vi "Read Counter.vi"(8 "error in (no error)":errorcluster, 10 "Params":variant, 11 "NI Counter Input in":refnum<class "NI Counter Input.lvclass">) -> (0 "error out":errorcluster, 2 "Data":variant, 3 "NI Counter Input out":refnum<class "NI Counter Input.lvclass">)   [LabVIEW 2020, in "NI DAQmx.lvlib" / "NI Counter Input.lvclass"]
uses:
  NI Counter Input.lvclass
  D:/WSGitHub/RTFWK/Realization/NI DAQmx Base/NI DAQmx Base.lvclass
  <vilib>/DAQmx/read.llb/DAQmx Read (Counter 1D DBL 1Chan NSamp).vi
  <vilib>/DAQmx/miscellaneous.llb/DAQmx Fill In Error Info.vi
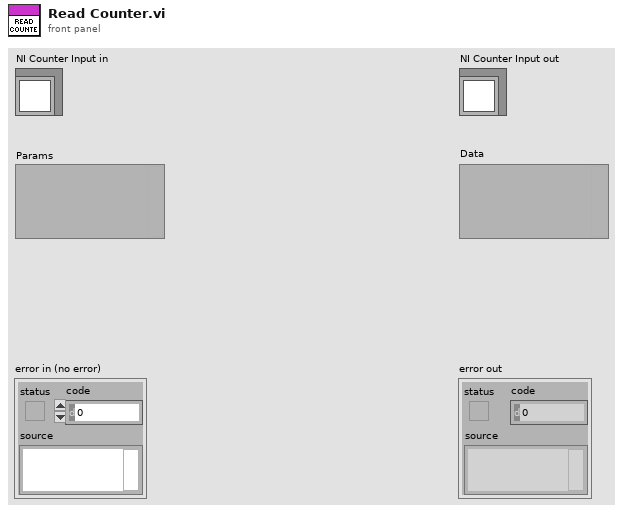
[diagram p1: front panel]
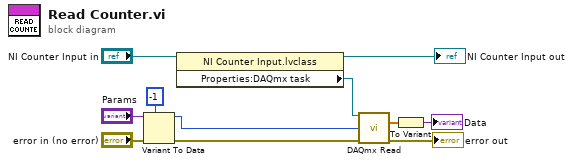
[diagram p0: block diagram]
diagram:
  n1 = Variant To Data(error in="error in (no error)", type=-1 ("number of samples per channel"), Variant="Params") -> (data=w1:i32, error out=w4:errorcluster)
  n2 = property class="NI Counter Input.lvclass"(reference="NI Counter Input in") -> (reference out=→"NI Counter Input out":refnum<class "NI Counter Input.lvclass">, "Properties:DAQmx task"=w6:refnum<k21>)  [unwired: 1 in, 1 out]
  n3 = call-poly <vilib>:"DAQmx Read.vi"("task/channels in"=w6, "number of samples per channel"=w1, "error in"=w4) -> ("data"=w8:dbl[], "error out"=→"error out":errorcluster)  [unwired: 10 in, 1 out]
  n4 = To Variant(anything=w8) -> (Variant=→"Data":variant)
